vi "First.vi"(8 "Error In":errorcluster, 10 "Known Host In":refnum<class "Known Host.lvclass">, 11 "KnownHosts In":refnum<class "Known Hosts.lvclass">) -> (0 "Error Out":errorcluster, 1 "Result":T1 items=["Success", "End of Hosts"], 2 "Known Host Out":refnum<class "Known Host.lvclass">, 3 "KnownHosts Out":refnum<class "Known Hosts.lvclass">)   [LabVIEW 2018, in "Toolkit.lvlib" / "Known Hosts.lvclass"]
uses:
  Known Hosts.lvclass
  Known Host/Known Host.lvclass
  Typedefs/Get Results.ctl
  Known Hosts.lvclass/Known Hosts.ctl
  Known Host/Known Host.lvclass/Known Host.ctl
  Session/Session.lvclass/Session.ctl
  SSH/SSH.lvclass/SSH.ctl
  Toolkit.lvlib
  Session/Session.lvclass
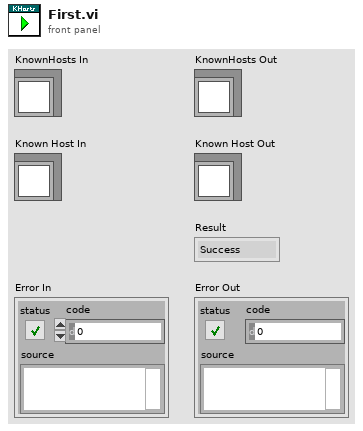
[diagram p1: front panel]
types:
  T1 = typedef "Toolkit.lvlib/Known Hosts.lvclass/Get Results.ctl" = i32
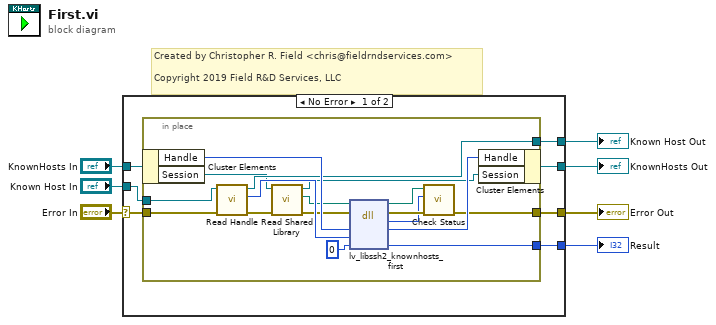
[diagram p0: block diagram]
diagram:
  # "Created by Christopher R. Field <chris@fieldrndservices.com>\n\nCopyright 2019 Field R&D Services, LLC"
  n1 = case shown="No Error" "Error In" {
    selector: "Error In" -> [w12 w34]
    tunnel: "KnownHosts In" -> [w14 w33]
    tunnel: [w11 w34] -> w5
    tunnel: [w13 w33] -> w4
    tunnel: "Known Host In" -> [w10 w32]
    tunnel: [w9 w32] -> w2
    tunnel: [w8 _] -> w1
    frame No Error {
      n2 = in-place {
        in-place-border: w12 -> [w24]
        in-place-border: [w27] -> w11
        in-place-border: w10 -> [w25]
        in-place-border: [w21] -> w9
        in-place-border: [w15] -> w8
        n3 = in-place-cluster #1(w14) -> ("Handle"=w31:u64, "Session"=w18:refnum<class "Session.lvclass">)
        n4 = call "Read Handle.vi"("Error In"=w24, "Known Host In"=w25) -> ("Error Out"=w23:errorcluster, "Handle"=w22:u64, "Known Host Out"=w21:refnum<class "Known Host.lvclass">)  [unwired: 7 in]
        n5 = call "Read Shared Library.vi"("Error In"=w23, "Session In"=w18) -> ("Erorr Out"=w19:errorcluster, "libssh2lv Shared Library"=w16:path, "Session Out"=w17:refnum<class "Session.lvclass">)  [unwired: 7 in]
        n6 = dll-call lib="lv-libssh2.*" fn="lv_libssh2_knownhosts_first"(path in=w16, error in=w19, "handle"=w31, "host"=w22, "result"=0) -> (path out=w28:path, error out=w29:errorcluster, "status"=w26:i32, "handle"=w30:u64, "result"=w15:i32)  [unwired: 2 in]
        n7 = call "Check Status.vi"("Error In"=w29, "Status"=w26, "lv-libssh2 Shared Library In"=w28) -> ("Error Out"=w27:errorcluster)  [unwired: 7 in, 1 out]
        n8 = in-place-cluster #1("Handle"=w30, "Session"=w17) -> (w13:refnum<class "Known Hosts.lvclass">)
      }
    }
    frame Error {
    }
  }
  "Error Out" <- w5
  "KnownHosts Out" <- w4
  "Known Host Out" <- w2
  "Result" <- w1
